vi "Set Defaults.vi"(11 "User in":refnum<class "User.lvclass">) -> (3 "User out":refnum<class "User.lvclass">)   [LabVIEW 2022 SP3, in "Test.lvlib" / "User.lvclass"]
uses:
  User.lvclass
  User.lvclass/User.ctl
  <vilib>/IlluminatedG/IG Conditum/Conditum/Columns/String/String.lvclass
  <vilib>/IlluminatedG/IG Conditum/Conditum/Columns/Timestamp/Timestamp.lvclass
  <vilib>/IlluminatedG/IG Conditum/Conditum/Columns/Boolean/Boolean.lvclass
  <vilib>/IlluminatedG/IG Conditum/Conditum/Columns/Integer/Integer.lvclass
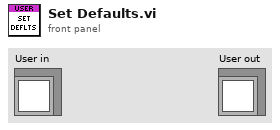
[diagram p1: front panel]
types:
  T1 = typedef "Test.lvlib/User.lvclass/Columns.ctl" = cluster{"Username":refnum<class "String.lvclass">, "Password":refnum<class "String.lvclass">, "Joined":refnum<class "Timestamp.lvclass">, "Last Activity":refnum<class "Timestamp.lvclass">, "Activated":refnum<class "Boolean.lvclass">, "Email":refnum<class "String.lvclass">, "Score":refnum<class "Integer.lvclass">}
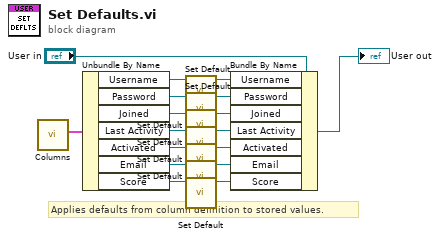
[diagram p0: block diagram]
diagram:
  # "Applies defaults from column definition to stored values."
  n1 = call "Columns.vi"() -> ("Columns"=w17:T1)  [unwired: 11 in]
  n2 = Unbundle By Name(w17) -> ("Username"=w16:refnum<class "String.lvclass">, "Password"=w14:refnum<class "String.lvclass">, "Joined"=w13:refnum<class "Timestamp.lvclass">, "Last Activity"=w12:refnum<class "Timestamp.lvclass">, "Activated"=w11:refnum<class "Boolean.lvclass">, "Email"=w10:refnum<class "String.lvclass">, "Score"=w15:refnum<class "Integer.lvclass">)
  n3 = call-dynamic "Set Default.vi"("String in"=w16) -> ("String out"=w9:refnum<class "String.lvclass">)  [unwired: 10 in]
  n4 = call-dynamic "Set Default.vi"("String in"=w14) -> ("String out"=w8:refnum<class "String.lvclass">)  [unwired: 10 in]
  n5 = call-dynamic "Set Default.vi"("Timestamp in"=w13) -> ("Timestamp out"=w7:refnum<class "Timestamp.lvclass">)  [unwired: 10 in]
  n6 = call-dynamic "Set Default.vi"("Timestamp in"=w12) -> ("Timestamp out"=w6:refnum<class "Timestamp.lvclass">)  [unwired: 10 in]
  n7 = call-dynamic "Set Default.vi"("Boolean in"=w11) -> ("Boolean out"=w5:refnum<class "Boolean.lvclass">)  [unwired: 10 in]
  n8 = call-dynamic "Set Default.vi"("String in"=w10) -> ("String out"=w4:refnum<class "String.lvclass">)  [unwired: 10 in]
  n9 = call-dynamic "Set Default.vi"("Integer in"=w15) -> ("Integer out"=w3:refnum<class "Integer.lvclass">)  [unwired: 10 in]
  n10 = Bundle By Name(cluster="User in", "Username"=w9, "Password"=w8, "Joined"=w7, "Last Activity"=w6, "Activated"=w5, "Email"=w4, "Score"=w3) -> (→"User out":refnum<class "User.lvclass">)
